vi "config.vi"(8 "error in (no error)":errorcluster, 11 "Impedancia":string(combo)="0") -> (0 "error out":errorcluster, 3 "DS360 out":refnum<class "DS360.lvclass">)   [LabVIEW 2019, in "DS360.lvclass"]
uses:
  DS360.lvclass
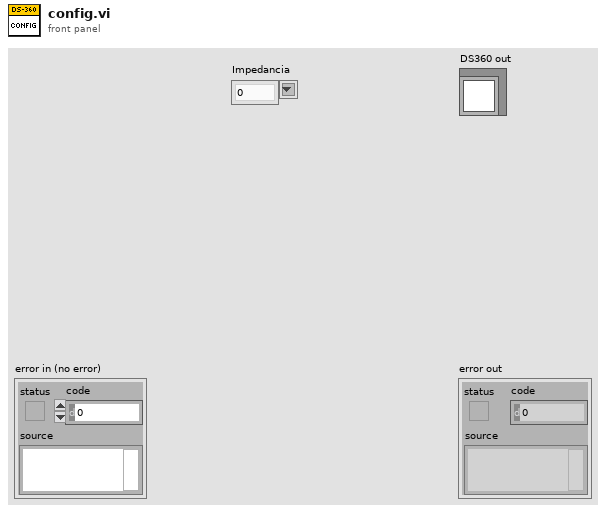
[diagram p1: front panel]
types:
  T1 = cluster{"error":bool, "code":i32, "source":string}
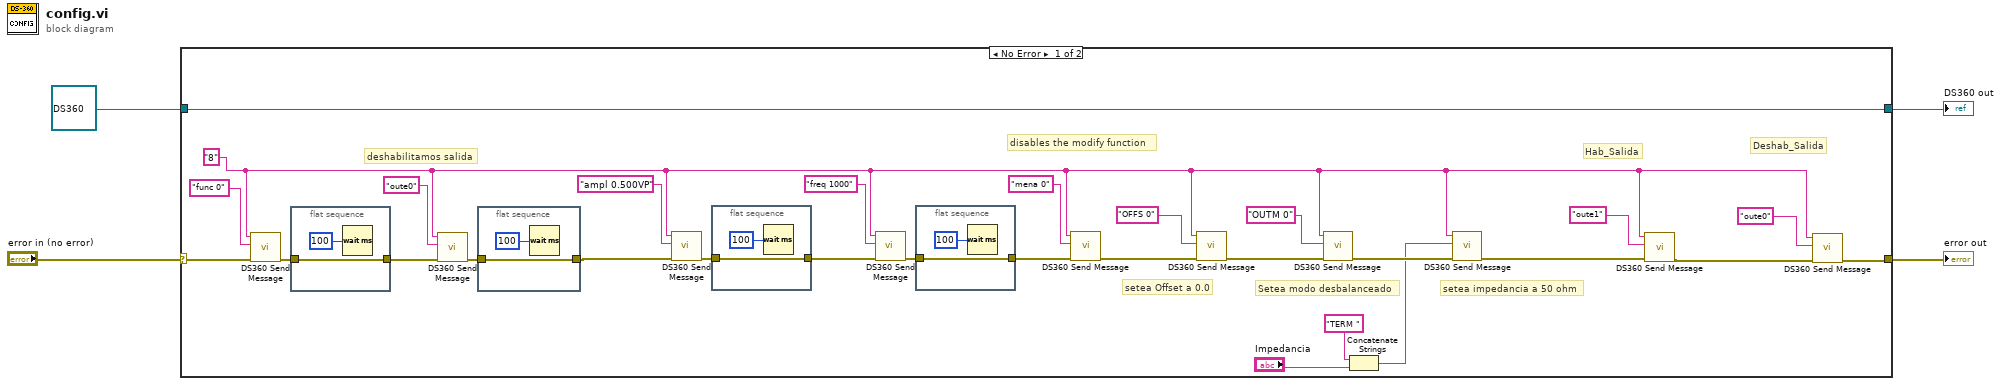
[diagram p0: block diagram]
diagram:
  n1 = case shown="No Error" "error in (no error)" {
    selector: "error in (no error)" -> [w27 w43]
    tunnel: [w15 w43] -> w3
    tunnel: [w33 w42] -> w1
    tunnel: refnum<class "DS360.lvclass"> refnum ("DS360 in") -> [w33 w42]
    frame No Error {
      w6 = "8" ("write buffer")
      # "setea impedancia a 50 ohm"
      # "Setea modo desbalanceado"
      # "setea Offset a 0.0"
      # "Deshab_Salida"
      # "Hab_Salida"
      # "disables the modify function"
      # "deshabilitamos salida"
      n2 = call <instrlib>:"DS360 Send Message.vi"("address string"=w6, "write buffer"="func 0", "error in"=w27) -> ("error out"=w30:T1)  [unwired: 3 in, 3 out]
      n3 = flat-sequence {
        tunnel: w30 -> [w41]
        tunnel: [w41] -> w29
        frame #0 {
          n4 = Wait (ms)(milliseconds to wait=u32 100) -> ()  [unwired: 1 out]
        }
      }
      n5 = call <instrlib>:"DS360 Send Message.vi"("address string"=w6, "write buffer"="oute0", "error in"=w29) -> ("error out"=w28:T1)  [unwired: 3 in, 3 out]
      n6 = flat-sequence {
        tunnel: w28 -> [w39]
        tunnel: [w39] -> w19
        frame #0 {
          n7 = Wait (ms)(milliseconds to wait=u32 100) -> ()  [unwired: 1 out]
        }
      }
      n8 = call <instrlib>:"DS360 Send Message.vi"("address string"=w6, "write buffer"="ampl 0.500VP", "error in"=w19) -> ("error out"=w23:T1)  [unwired: 3 in, 3 out]
      n9 = flat-sequence {
        tunnel: w23 -> [w37]
        tunnel: [w37] -> w22
        frame #0 {
          n10 = Wait (ms)(milliseconds to wait=u32 100) -> ()  [unwired: 1 out]
        }
      }
      n11 = call <instrlib>:"DS360 Send Message.vi"("address string"=w6, "write buffer"="freq 1000", "error in"=w22) -> ("error out"=w21:T1)  [unwired: 3 in, 3 out]
      n12 = flat-sequence {
        tunnel: w21 -> [w35]
        tunnel: [w35] -> w20
        frame #0 {
          n13 = Wait (ms)(milliseconds to wait=u32 100) -> ()  [unwired: 1 out]
        }
      }
      n14 = call <instrlib>:"DS360 Send Message.vi"("address string"=w6, "write buffer"="mena 0", "error in"=w20) -> ("error out"=w7:T1)  [unwired: 3 in, 3 out]
      n15 = call <instrlib>:"DS360 Send Message.vi"("address string"=w6, "write buffer"="OFFS 0", "error in"=w7) -> ("error out"=w13:T1)  [unwired: 3 in, 3 out]
      n16 = call <instrlib>:"DS360 Send Message.vi"("address string"=w6, "write buffer"="OUTM 0", "error in"=w13) -> ("error out"=w12:T1)  [unwired: 3 in, 3 out]
      n17 = Concatenate Strings("TERM " ("write buffer"), "Impedancia") -> (w8:string)
      n18 = call <instrlib>:"DS360 Send Message.vi"("address string"=w6, "write buffer"=w8, "error in"=w12) -> ("error out"=w5:T1)  [unwired: 3 in, 3 out]
      n19 = call <instrlib>:"DS360 Send Message.vi"("address string"=w6, "write buffer"="oute1", "error in"=w5) -> ("error out"=w16:T1)  [unwired: 3 in, 3 out]
      n20 = call <instrlib>:"DS360 Send Message.vi"("address string"=w6, "write buffer"="oute0", "error in"=w16) -> ("error out"=w15:T1)  [unwired: 3 in, 3 out]
    }
    frame Error {
    }
  }
  "error out" <- w3
  "DS360 out" <- w1
